vi "Angle Snap.vi"(10 "Enable?":bool) -> (1 "Gyro Steer?":bool, 3 "Heading Out":dbl)   [LabVIEW 2014]
uses:
  Common Code/Change Detect Boolean.vi
  Robot Global Data.vi
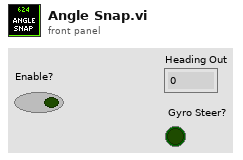
[diagram p1: front panel]
types:
  T1 = typedef "IMU Data.ctl" = cluster{"Pitch":sgl, "Roll":sgl, "Yaw":sgl, "Data Valid?":bool, "Temp":sgl, "MOVING":bool, "NAVX_CAL_STATUS":T2, "NAVX_OP_STATUS":T3, "YAW_STABLE":bool, "Accel X":sgl, "Accel Y":sgl, "Accel Z":sgl, "Accel Magnitude":sgl, "Pitch Rate":sgl, "Roll Rate":sgl, "Yaw Rate":sgl}
  T2 = typedef "navX-MXP IMU.lvlib/navX NAVX_CAL_STATUS.ctl" = u8
  T3 = typedef "navX-MXP IMU.lvlib/navX NAVX_OP_STATUS.ctl" = u8
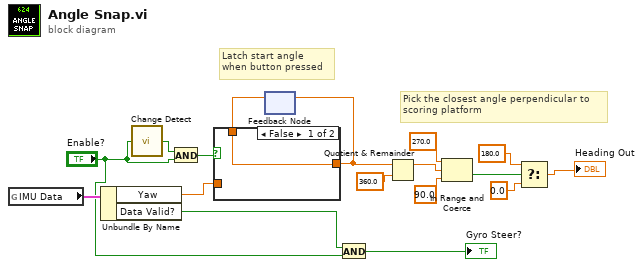
[diagram p0: block diagram]
diagram:
  # "Pick the closest angle perpendicular to\nscoring platform"
  # "Latch start angle\nwhen button pressed"
  n1 = global read "Robot Global Data.vi" "IMU Data"() -> (w17:T1)
  n2 = Unbundle By Name(w17) -> ("Yaw"=w14:sgl, "Data Valid?"=w3:bool)
  n3 = call-poly "Change Detect.vi"("In"="Enable?") -> ("Changed?"=w16:bool)
  n4 = And(x=w16, y="Enable?") -> (x .and. y?=w15:bool)
  n5 = feedback #1() -> (w13:sgl)  [unwired: 1 in]
  n6 = case shown="False" w15 {
    tunnel: w14 -> [_ w19]
    tunnel: [w18 w19] -> w12
    tunnel: w13 -> [w18 _]
    frame False {
    }
    frame True {
    }
  }
  n7 = feedback-in #1(w12) -> ()
  n8 = And(x=w3, y="Enable?") -> (x .and. y?=→"Gyro Steer?":bool)
  n9 = Quotient & Remainder(x=w12, y=sgl 360.0) -> (x-y*floor(x/y)=w10:sgl)  [unwired: 1 out]
  n10 = In Range and Coerce(upper limit=sgl 270.0, x=w10, lower limit=sgl 90.0) -> (In Range?=w7:bool)  [unwired: 1 out]
  n11 = Select(t=180.0, s=w7, f=0.0 ("t")) -> (s? t:f=→"Heading Out":dbl)
